vi "Input_Sensors_Drive.vi"() -> (3 "Drive Inputs":T2)   [LabVIEW 2012]
uses:
  Input_Sensors_Drive.ctl
  <vilib>/Rock Robotics/WPI/CAN/Jaguar/SubVIs/WPI_CANJaguar_SpeedReference.ctl
  <vilib>/Rock Robotics/WPI/CAN/Jaguar/SubVIs/WPI_CANJaguar_StatusSelect.ctl
panel:
  out "Speed Reference 4":T1 items=["Encoder"=0, "Inv Encoder"=2, "Quad Encoder"=3, "None"=255]
  out "Speed Reference 3":T1 items=["Encoder"=0, "Inv Encoder"=2, "Quad Encoder"=3, "None"=255]
  out "Speed Reference 2":T1 items=["Encoder"=0, "Inv Encoder"=2, "Quad Encoder"=3, "None"=255]
  out "Speed Reference 1":T1 items=["Encoder"=0, "Inv Encoder"=2, "Quad Encoder"=3, "None"=255]
  out "error out":errorcluster
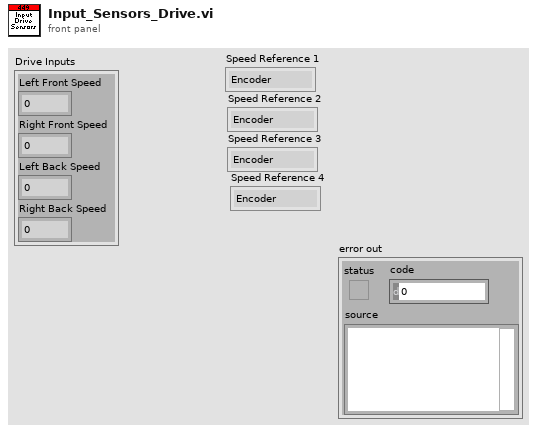
[diagram p1: front panel]
types:
  T1 = typedef "WPI_CANJaguar_SpeedReference.ctl" = u8
  T2 = typedef "Input_Sensors_Drive.ctl" = cluster{"Left Front Speed":dbl, "Right Front Speed":dbl, "Left Back Speed":dbl, "Right Back Speed":dbl}
  T3 = typedef "WPI_CANJaguar_StatusSelect.ctl" = enum16{"Output Percent VBus", "Output Voltage", "Bus Voltage", "Current", "Temperature", "Position", "Speed", "Limit Switches", "Faults", "Fault Counters", "Power Cycle"}
  T4 = typedef "WPI_MotorControlDeviceRef.ctl" = cluster{"DeviceStatus":errorcluster, "Type":enum16{"PWM", "CAN"}, "PWM":cluster{"Digital Module":T5, "PWM Channel":T6, "DeadBand":T7}, "CAN":cluster{"Device Number":u8, "Control Mode":T8, "Semaphore":T9, "Max Vout":dbl}, "Invert":bool, "TransformRef":T10, "InvTransformRef":T10}
  T5 = typedef "FPGA_TypedefDigitalModule.ctl" = enum16{"Digital Module 1", "Digital Module 2"}
  T6 = typedef "FPGA_DIOPWMChannel.ctl" = enum8{"PWM 1", "PWM 2", "PWM 3", "PWM 4", "PWM 5", "PWM 6", "PWM 7", "PWM 8", "PWM 9", "PWM 10", "Invalid"}
  T7 = typedef "WPI_PWMDeadband.ctl" = cluster{"Name":string, "maxPositivePwm":i32, "minPositivePwm":i32, "centerPwm":i32, "maxNegativePwm":i32, "minNegativePwm":i32, "angularRange":u16}
  T8 = typedef "WPI_CANJaguar_ControlMode.ctl" = enum8{"Percent VBus", "Current", "Speed", "Position", "Voltage"}
  T9 = typedef "Semaphore RefNum" = refnum<k1>
  T10 = typedef "WPI_PWMTransform_ConPane.ctl" = refnum<vi>
  T11 = typedef "WPI_CANJaguar_Status.ctl" = cluster{"Output Percent VBus":dbl, "Output Voltage":dbl, "Bus Voltage":dbl, "Current":dbl, "Temperature":dbl, "Position":dbl, "Speed":dbl, "Limits":cluster{"Forward Limit":bool, "Reverse Limit":bool, "Forward Soft Limit":bool, "Reverse Soft Limit":bool, "Sticky Forward Limit":bool, "Sticky Reverse Limit":bool, "Sticky Forward Soft Limit":bool, "Sticky Reverse Soft Limit":bool}, "Faults":cluster{"Current Fault":bool, "Temperature Fault":bool, "Bus Voltage Fault":bool, "Gate Driver Fault":bool, "Comm Fault":bool}, "Fault Counters":cluster{"Current Faults":u8, "Temperature Faults":u8, "Bus Voltage Faults":u8, "Gate Driver Faults":u8, "Comm Faults":u8, "CAN Status":u8, "CAN RX Errors":u8, "CAN TX Errors":u8}, "Power Cycle":bool}
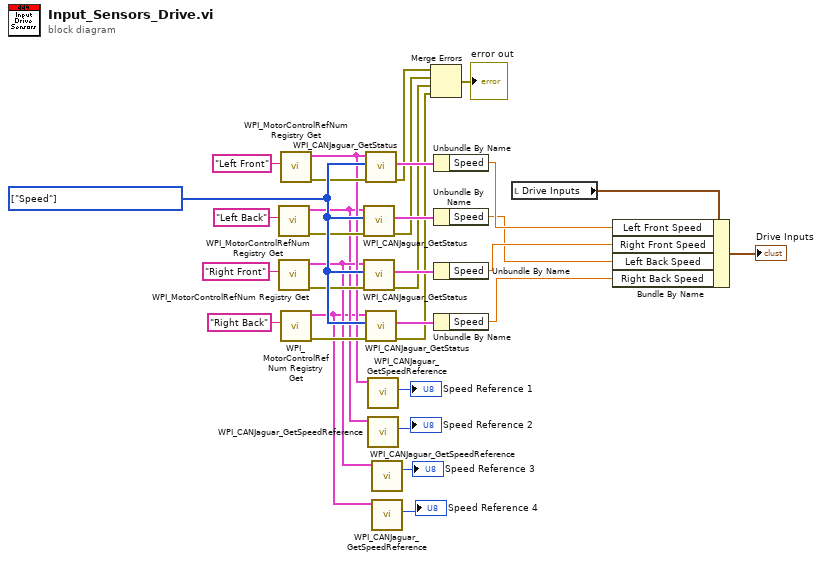
[diagram p0: block diagram]
diagram:
  w28 = T3[] [enum."Speed"] items=["Output Percent VBus", "Output Voltage", "Bus Voltage", "Current", "Temperature", "Position", "Speed", "Limit Switches", "Faults", "Fault Counters", "Power Cycle"] ("Status Select")
  n1 = call <vilib>:"WPI_MotorControlRefNum Registry Get.vi"("refnum name"="Left Back") -> ("error out"=w11:errorcluster, "MotorControlDevRef"=w6:T4)  [unwired: 9 in]
  n2 = call <vilib>:"WPI_MotorControlRefNum Registry Get.vi"("refnum name"="Right Front") -> ("error out"=w15:errorcluster, "MotorControlDevRef"=w7:T4)  [unwired: 9 in]
  n3 = call <vilib>:"WPI_MotorControlRefNum Registry Get.vi"("refnum name"="Left Front") -> ("error out"=w13:errorcluster, "MotorControlDevRef"=w8:T4)  [unwired: 9 in]
  n4 = call <vilib>:"WPI_MotorControlRefNum Registry Get.vi"("refnum name"="Right Back") -> ("error out"=w9:errorcluster, "MotorControlDevRef"=w5:T4)  [unwired: 9 in]
  n5 = call <vilib>:"WPI_CANJaguar_GetStatus.vi"("error in (no error)"=w11, "Status Select"=w28, "CAN Jaguar Ref"=w6) -> ("error out"=w20:errorcluster, "Status"=w31:T11)  [unwired: 6 in, 1 out]
  n6 = call <vilib>:"WPI_CANJaguar_GetStatus.vi"("error in (no error)"=w15, "Status Select"=w28, "CAN Jaguar Ref"=w7) -> ("error out"=w19:errorcluster, "Status"=w30:T11)  [unwired: 6 in, 1 out]
  n7 = call <vilib>:"WPI_CANJaguar_GetStatus.vi"("error in (no error)"=w13, "Status Select"=w28, "CAN Jaguar Ref"=w8) -> ("error out"=w21:errorcluster, "Status"=w32:T11)  [unwired: 6 in, 1 out]
  n8 = call <vilib>:"WPI_CANJaguar_GetStatus.vi"("error in (no error)"=w9, "Status Select"=w28, "CAN Jaguar Ref"=w5) -> ("error out"=w18:errorcluster, "Status"=w29:T11)  [unwired: 6 in, 1 out]
  n9 = call <vilib>:"WPI_CANJaguar_GetSpeedReference.vi"("CAN Jaguar Ref"=w8) -> ("Speed Reference"=→"Speed Reference 1":T1)  [unwired: 8 in, 2 out]
  n10 = call <vilib>:"WPI_CANJaguar_GetSpeedReference.vi"("CAN Jaguar Ref"=w6) -> ("Speed Reference"=→"Speed Reference 2":T1)  [unwired: 8 in, 2 out]
  n11 = call <vilib>:"WPI_CANJaguar_GetSpeedReference.vi"("CAN Jaguar Ref"=w7) -> ("Speed Reference"=→"Speed Reference 3":T1)  [unwired: 8 in, 2 out]
  n12 = call <vilib>:"WPI_CANJaguar_GetSpeedReference.vi"("CAN Jaguar Ref"=w5) -> ("Speed Reference"=→"Speed Reference 4":T1)  [unwired: 8 in, 2 out]
  n13 = Merge Errors(w21, w20, w19, w18) -> (→"error out":errorcluster)
  n14 = Unbundle By Name(w32) -> ("Speed"=w26:dbl)
  n15 = Unbundle By Name(w31) -> ("Speed"=w24:dbl)
  n16 = Unbundle By Name(w30) -> ("Speed"=w25:dbl)
  n17 = Unbundle By Name(w29) -> ("Speed"=w23:dbl)
  n18 = local read "Drive Inputs"() -> (w27:T2)
  n19 = Bundle By Name(cluster=w27, "Left Front Speed"=w26, "Right Front Speed"=w25, "Left Back Speed"=w24, "Right Back Speed"=w23) -> (→"Drive Inputs":T2)
